vi "FPGA myRIO Ultrasound (1) (1).vi"() -> ()   [LabVIEW 2015]
uses:
  <vilib>/rvi/Emulation/niFpgaGetClockAttributes.vi
  <vilib>/rvi/Emulation/niFpgaSctlEmulationGetInTimedLoop.vi
  <vilib>/rvi/Emulation/niFpgaEmulationReportErrorSimple.vi
  <vilib>/rvi/eio/common/nirviEmuTemplateMethod_errors.vi
  <vilib>/rvi/Emulation/niFpgaCriticalErrorInLSC.vi
  <vilib>/rvi/Emulation/niFpgaProcessEmulError.vi
  <vilib>/eio/EIONode/EIONode.xnode
panel:
  in  "Trigger pulse interval (mSec) 4":u32=200
  out "Time of flight (uS) 4":u32
  out "Distance (cm) 4":sgl
  out "Distance (m) 4":sgl
  in  "Trigger pulse interval (mSec) 3":u32=200
  out "Time of flight (uS) 3":u32
  out "Distance (cm) 3":sgl
  out "Distance (m) 3":sgl
  in  "Trigger pulse interval (mSec) 2":u32=200
  out "Time of flight (uS) 2":u32
  out "Distance (cm) 2":sgl
  out "Distance (m) 2":sgl
  out "Distance (m)":sgl
  out "Distance (cm)":sgl
  in  "Trigger pulse interval (mSec)":u32=200
  out "Time of flight (uS)":u32
  in  "stop":bool
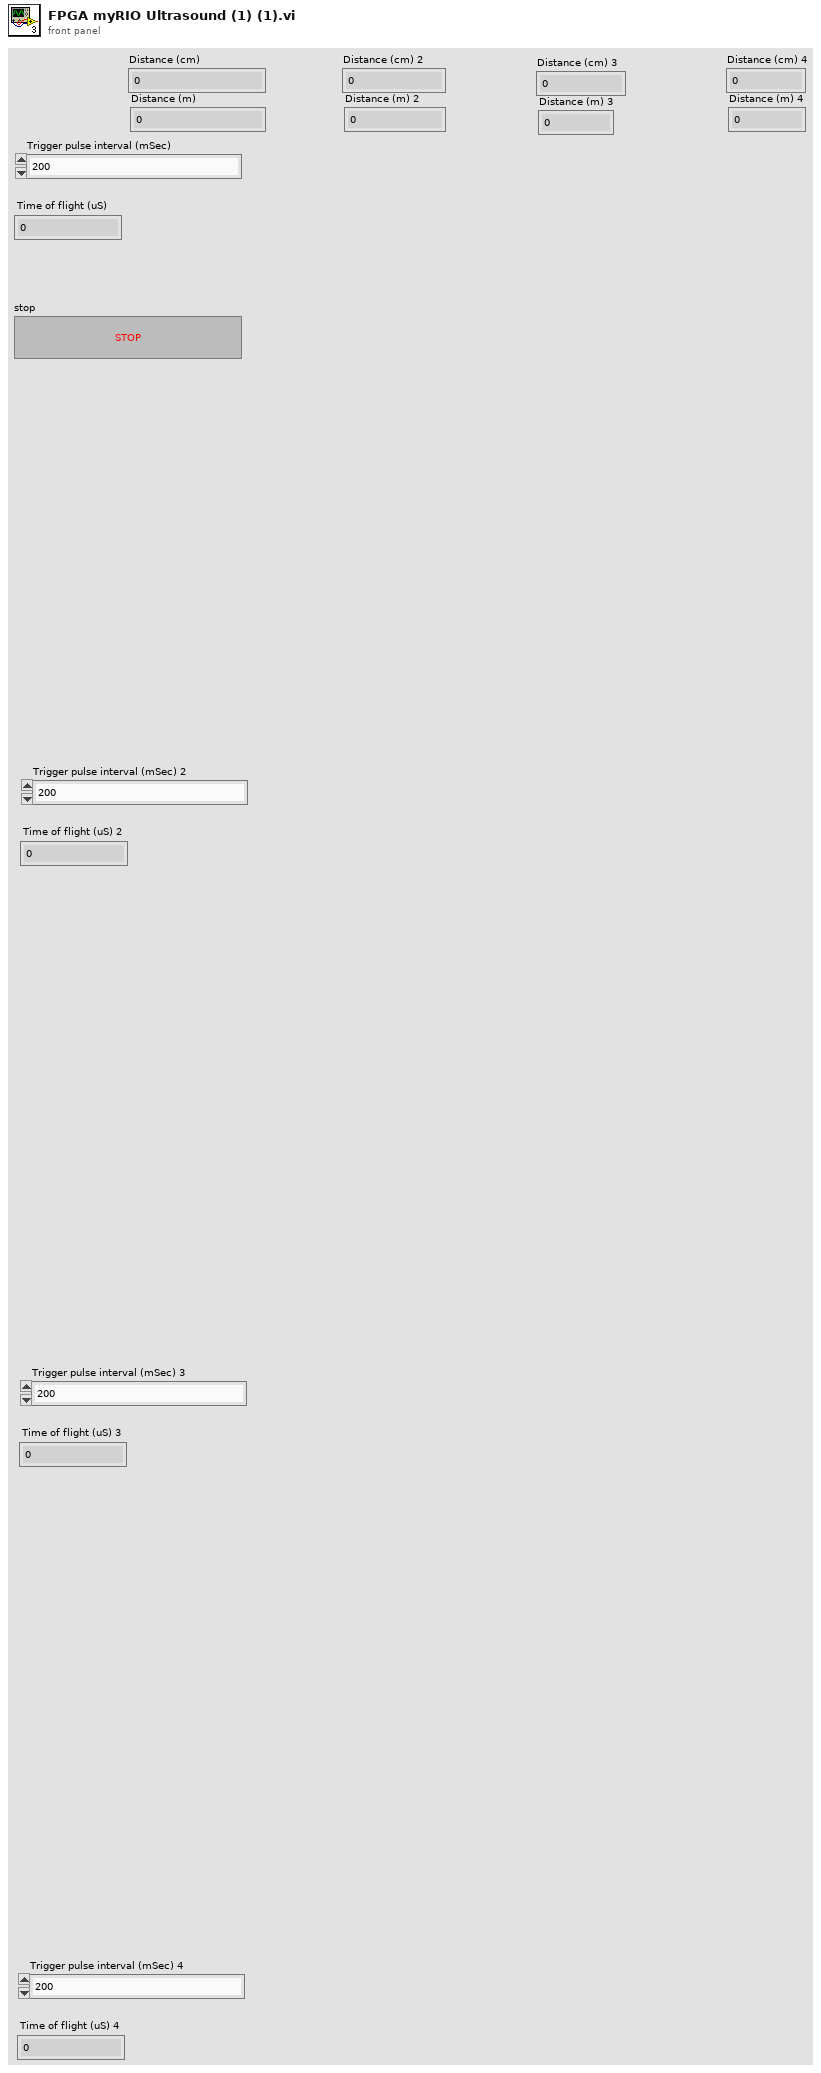
[diagram p1: front panel]
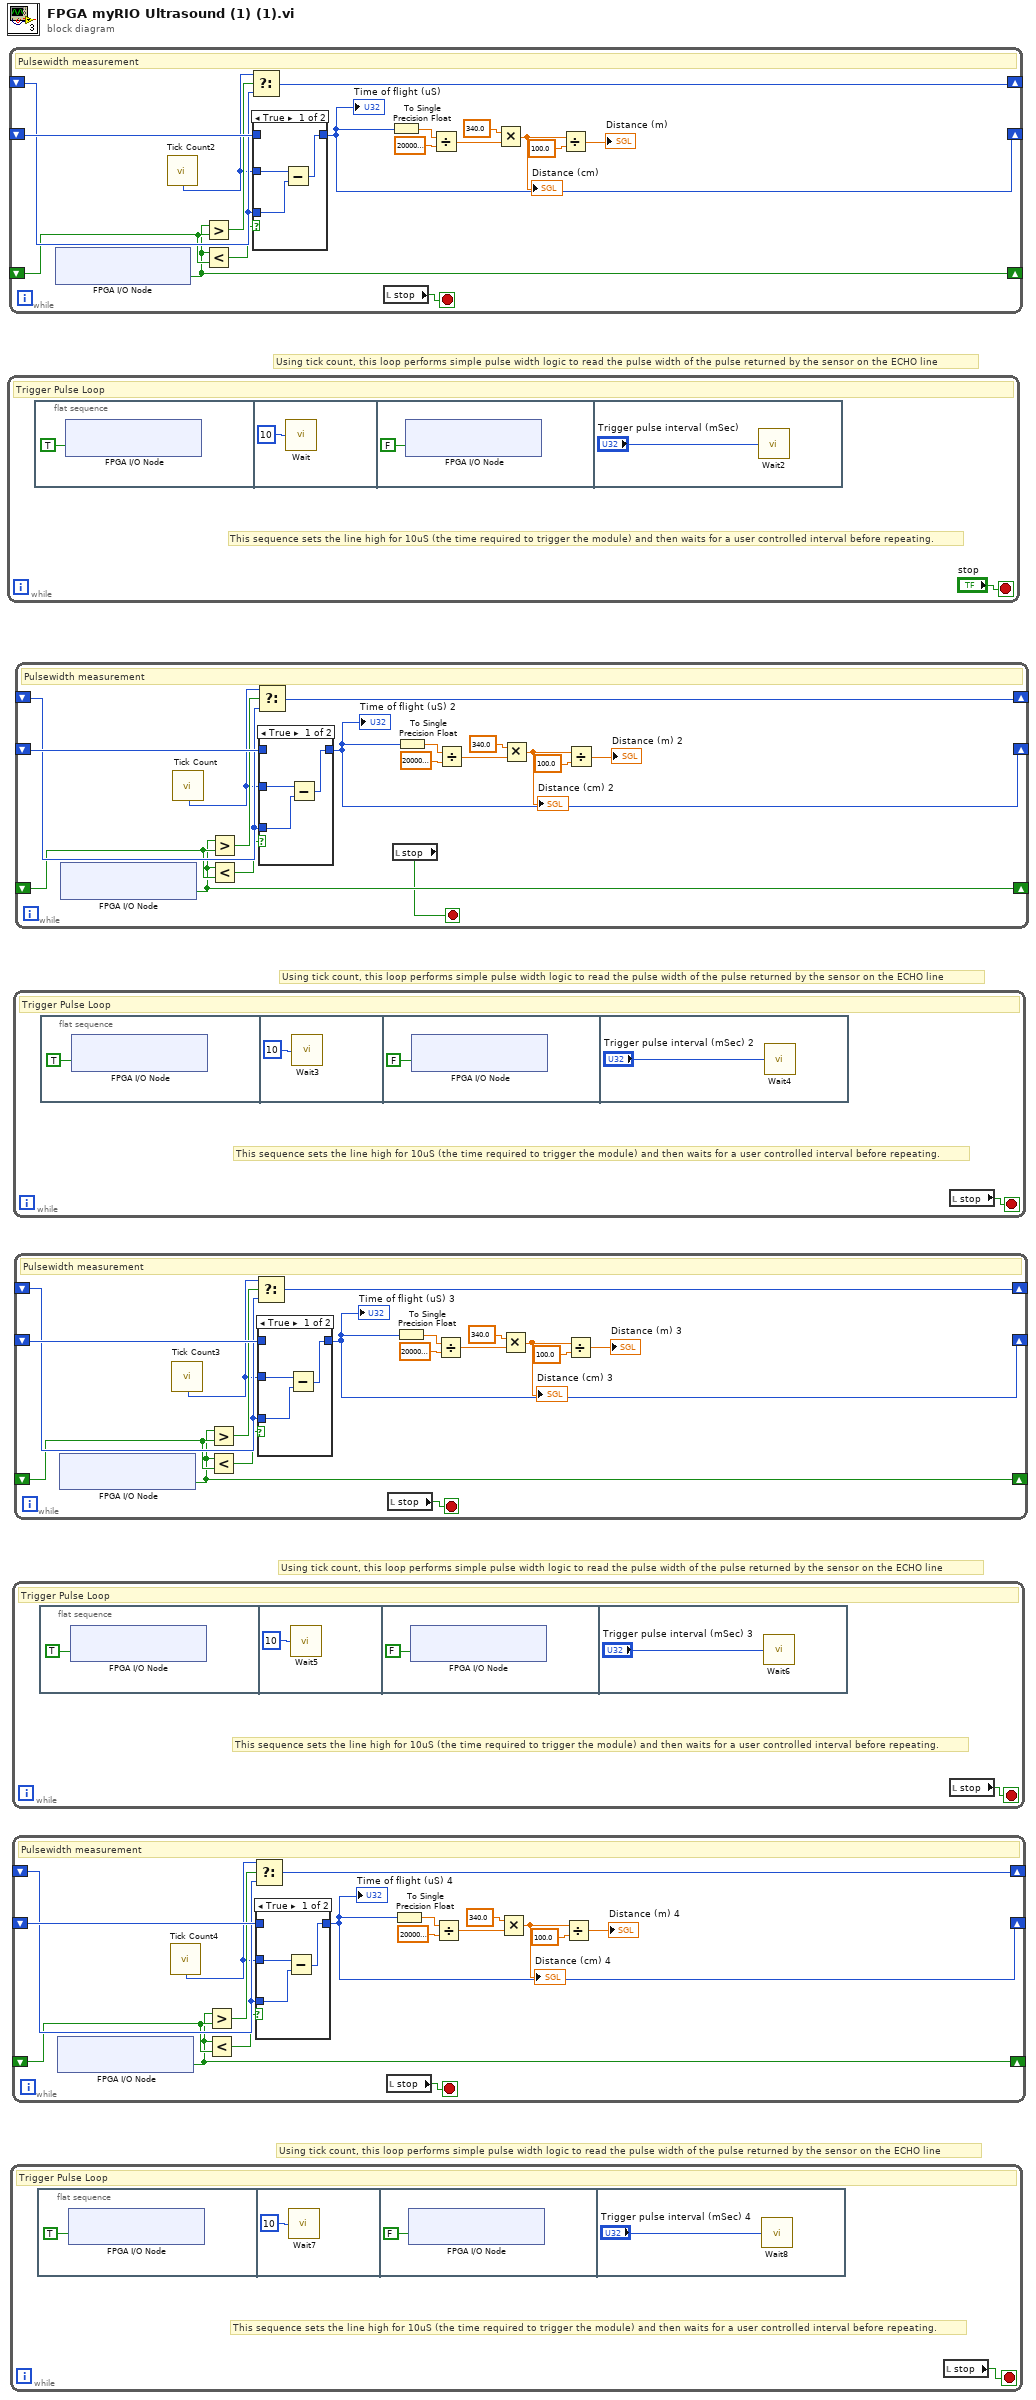
[diagram p0: block diagram]
diagram:
  # "Using tick count, this loop performs simple pulse width logic to read the pulse width of the pulse returned by the sensor on the ECHO line"
  # "Using tick count, this loop performs simple pulse width logic to read the pulse width of the pulse returned by the sensor on the ECHO line"
  # "Using tick count, this loop performs simple pulse width logic to read the pulse width of the pulse returned by the sensor on the ECHO line"
  # "Using tick count, this loop performs simple pulse width logic to read the pulse width of the pulse returned by the sensor on the ECHO line"
  n1 = while {
    stop <- "stop" stop-if-true
    # "This sequence sets the line high for 10uS (the time required to trigger the module) and then waits for a user controlled interval before repeating."
    # "Trigger Pulse Loop"
    n2 = flat-sequence {
      frame #0 {
        n3 = xnode "FPGA I/O Node"("ConnectorB/DIO7"=TRUE ("ConnectorC/DIO6")) -> ()  [unwired: 1 in, 1 out]
      }
      frame #1 {
        n4 = call "Wait"("Count(uSec)"=u32 10) -> ()  [unwired: 1 out]
      }
      frame #2 {
        n5 = xnode "FPGA I/O Node"("ConnectorB/DIO7"=FALSE ("ConnectorC/DIO6")) -> ()  [unwired: 1 in, 1 out]
      }
      frame #3 {
        n6 = call "Wait2"("Count(mSec)"="Trigger pulse interval (mSec)") -> ()  [unwired: 1 out]
      }
    }
  }
  n7 = while "Pulsewidth Measurement + Sound Output" {
    shift-left: _ -> [w22]
    shift-right: [w13] -> _
    shift-left: _ -> [w21]
    shift-right: [w20] -> _
    shift-left: _ -> [w18]
    shift-right: [w16] -> _
    stop <- w14 stop-if-true
    # "Pulsewidth measurement"
    n8 = xnode "FPGA I/O Node"() -> ("ConnectorB/DIO3"=w16:bool)  [unwired: 1 in, 1 out]
    n9 = call "Tick Count2"() -> ("Tick Count(uSec)"=w15:u32)
    n10 = Greater?(x=w16, y=w18) -> (0:w19:bool)
    n11 = Less?(x=w16, y=w18) -> (x < y?=w17:bool)
    n12 = Select(t=w15, s=w19, f=w21) -> (s? t:f=w20:u32)
    n13 = case shown="True" w17 {
      tunnel: w22 -> [_ w26]
      tunnel: w15 -> [w23 _]
      tunnel: w21 -> [w24 _]
      tunnel: [w25 w26] -> w13
      frame True {
        n14 = Subtract(x=w23, y=w24) -> (x-y=w25:u32)
      }
      frame False {
      }
    }
    "Time of flight (uS)" <- w13
    n15 = local read "stop"() -> (w14:bool)
    n16 = To Single Precision Float(number=w13) -> (single precision float=w12:sgl)
    n17 = Divide(x=w12, y=sgl 20000000.0) -> (x/y=w10:sgl)
    n18 = Multiply(x=sgl 340.0, y=w10) -> (x*y=w8:sgl)
    "Distance (cm)" <- w8
    n19 = Divide(x=w8, y=sgl 100.0) -> (x/y=→"Distance (m)":sgl)
  }
  n20 = while {
    stop <- w27 stop-if-true
    # "This sequence sets the line high for 10uS (the time required to trigger the module) and then waits for a user controlled interval before repeating."
    # "Trigger Pulse Loop"
    n21 = flat-sequence {
      frame #0 {
        n22 = xnode "FPGA I/O Node"("ConnectorB/DIO4"=TRUE ("ConnectorC/DIO6")) -> ()  [unwired: 1 in, 1 out]
      }
      frame #1 {
        n23 = call "Wait7"("Count(uSec)"=u32 10) -> ()  [unwired: 1 out]
      }
      frame #2 {
        n24 = xnode "FPGA I/O Node"("ConnectorB/DIO4"=FALSE ("ConnectorC/DIO6")) -> ()  [unwired: 1 in, 1 out]
      }
      frame #3 {
        n25 = call "Wait8"("Count(mSec)"="Trigger pulse interval (mSec) 4") -> ()  [unwired: 1 out]
      }
    }
    n26 = local read "stop"() -> (w27:bool)
  }
  n27 = while {
    stop <- w32 stop-if-true
    # "This sequence sets the line high for 10uS (the time required to trigger the module) and then waits for a user controlled interval before repeating."
    # "Trigger Pulse Loop"
    n28 = flat-sequence {
      frame #0 {
        n29 = xnode "FPGA I/O Node"("ConnectorB/DIO5"=TRUE ("ConnectorC/DIO6")) -> ()  [unwired: 1 in, 1 out]
      }
      frame #1 {
        n30 = call "Wait5"("Count(uSec)"=u32 10) -> ()  [unwired: 1 out]
      }
      frame #2 {
        n31 = xnode "FPGA I/O Node"("ConnectorB/DIO5"=FALSE ("ConnectorC/DIO6")) -> ()  [unwired: 1 in, 1 out]
      }
      frame #3 {
        n32 = call "Wait6"("Count(mSec)"="Trigger pulse interval (mSec) 3") -> ()  [unwired: 1 out]
      }
    }
    n33 = local read "stop"() -> (w32:bool)
  }
  n34 = while "Pulsewidth Measurement + Sound Output" {
    shift-left: _ -> [w53]
    shift-right: [w44] -> _
    shift-left: _ -> [w52]
    shift-right: [w51] -> _
    shift-left: _ -> [w49]
    shift-right: [w47] -> _
    stop <- w45 stop-if-true
    # "Pulsewidth measurement"
    n35 = xnode "FPGA I/O Node"() -> ("ConnectorB/DIO0"=w47:bool)  [unwired: 1 in, 1 out]
    n36 = call "Tick Count4"() -> ("Tick Count(uSec)"=w46:u32)
    n37 = Greater?(x=w47, y=w49) -> (0:w50:bool)
    n38 = Less?(x=w47, y=w49) -> (x < y?=w48:bool)
    n39 = Select(t=w46, s=w50, f=w52) -> (s? t:f=w51:u32)
    n40 = case shown="True" w48 {
      tunnel: w53 -> [_ w57]
      tunnel: w46 -> [w54 _]
      tunnel: w52 -> [w55 _]
      tunnel: [w56 w57] -> w44
      frame True {
        n41 = Subtract(x=w54, y=w55) -> (x-y=w56:u32)
      }
      frame False {
      }
    }
    "Time of flight (uS) 4" <- w44
    n42 = local read "stop"() -> (w45:bool)
    n43 = To Single Precision Float(number=w44) -> (single precision float=w43:sgl)
    n44 = Divide(x=w43, y=sgl 20000000.0) -> (x/y=w41:sgl)
    n45 = Multiply(x=sgl 340.0, y=w41) -> (x*y=w39:sgl)
    "Distance (cm) 4" <- w39
    n46 = Divide(x=w39, y=sgl 100.0) -> (x/y=→"Distance (m) 4":sgl)
  }
  n47 = while {
    stop <- w58 stop-if-true
    # "This sequence sets the line high for 10uS (the time required to trigger the module) and then waits for a user controlled interval before repeating."
    # "Trigger Pulse Loop"
    n48 = flat-sequence {
      frame #0 {
        n49 = xnode "FPGA I/O Node"("ConnectorB/DIO6"=TRUE ("ConnectorC/DIO6")) -> ()  [unwired: 1 in, 1 out]
      }
      frame #1 {
        n50 = call "Wait3"("Count(uSec)"=u32 10) -> ()  [unwired: 1 out]
      }
      frame #2 {
        n51 = xnode "FPGA I/O Node"("ConnectorB/DIO6"=FALSE ("ConnectorC/DIO6")) -> ()  [unwired: 1 in, 1 out]
      }
      frame #3 {
        n52 = call "Wait4"("Count(mSec)"="Trigger pulse interval (mSec) 2") -> ()  [unwired: 1 out]
      }
    }
    n53 = local read "stop"() -> (w58:bool)
  }
  n54 = while "Pulsewidth Measurement + Sound Output" {
    shift-left: _ -> [w79]
    shift-right: [w71] -> _
    shift-left: _ -> [w78]
    shift-right: [w77] -> _
    shift-left: _ -> [w75]
    shift-right: [w73] -> _
    stop <- w63 stop-if-true
    # "Pulsewidth measurement"
    n55 = xnode "FPGA I/O Node"() -> ("ConnectorB/DIO1"=w73:bool)  [unwired: 1 in, 1 out]
    n56 = call "Tick Count3"() -> ("Tick Count(uSec)"=w72:u32)
    n57 = Greater?(x=w73, y=w75) -> (0:w76:bool)
    n58 = Less?(x=w73, y=w75) -> (x < y?=w74:bool)
    n59 = Select(t=w72, s=w76, f=w78) -> (s? t:f=w77:u32)
    n60 = case shown="True" w74 {
      tunnel: w79 -> [_ w83]
      tunnel: w72 -> [w80 _]
      tunnel: w78 -> [w81 _]
      tunnel: [w82 w83] -> w71
      frame True {
        n61 = Subtract(x=w80, y=w81) -> (x-y=w82:u32)
      }
      frame False {
      }
    }
    "Time of flight (uS) 3" <- w71
    n62 = local read "stop"() -> (w63:bool)
    n63 = To Single Precision Float(number=w71) -> (single precision float=w70:sgl)
    n64 = Divide(x=w70, y=sgl 20000000.0) -> (x/y=w68:sgl)
    n65 = Multiply(x=sgl 340.0, y=w68) -> (x*y=w66:sgl)
    "Distance (cm) 3" <- w66
    n66 = Divide(x=w66, y=sgl 100.0) -> (x/y=→"Distance (m) 3":sgl)
  }
  n67 = while "Pulsewidth Measurement + Sound Output" {
    shift-left: _ -> [w100]
    shift-right: [w92] -> _
    shift-left: _ -> [w99]
    shift-right: [w98] -> _
    shift-left: _ -> [w96]
    shift-right: [w94] -> _
    stop <- w84 stop-if-true
    # "Pulsewidth measurement"
    n68 = xnode "FPGA I/O Node"() -> ("ConnectorB/DIO2"=w94:bool)  [unwired: 1 in, 1 out]
    n69 = call "Tick Count"() -> ("Tick Count(uSec)"=w93:u32)
    n70 = Greater?(x=w94, y=w96) -> (0:w97:bool)
    n71 = Less?(x=w94, y=w96) -> (x < y?=w95:bool)
    n72 = Select(t=w93, s=w97, f=w99) -> (s? t:f=w98:u32)
    n73 = case shown="True" w95 {
      tunnel: w100 -> [_ w104]
      tunnel: w93 -> [w101 _]
      tunnel: w99 -> [w102 _]
      tunnel: [w103 w104] -> w92
      frame True {
        n74 = Subtract(x=w101, y=w102) -> (x-y=w103:u32)
      }
      frame False {
      }
    }
    "Time of flight (uS) 2" <- w92
    n75 = local read "stop"() -> (w84:bool)
    n76 = To Single Precision Float(number=w92) -> (single precision float=w91:sgl)
    n77 = Divide(x=w91, y=sgl 20000000.0) -> (x/y=w89:sgl)
    n78 = Multiply(x=sgl 340.0, y=w89) -> (x*y=w87:sgl)
    "Distance (cm) 2" <- w87
    n79 = Divide(x=w87, y=sgl 100.0) -> (x/y=→"Distance (m) 2":sgl)
  }
